vi "Demo v4_QL.vi"() -> ()   [LabVIEW 2013]
panel:
  out "0, 1":i16[](graph)
  out "Out of bound":bool
  out "Hit tube":bool
  out "Unrolled state":i32
  out "Numeric":i32
  out "Iteration":i32
  out "Q":dbl[][](array[numeric])
  in  "Slow":bool=TRUE
  out "sum":dbl
  in  "Reset Q":bool
  in  "stop":bool
  out "JUMP?":bool
  out "SCORE":i32
  out "FAIL!":bool
  in  "a":dbl=-0.3
  in  "Jump speed":dbl=3.0
  out "Picture":i32[][](graph)
  # "JUMP"
  # "FALL"
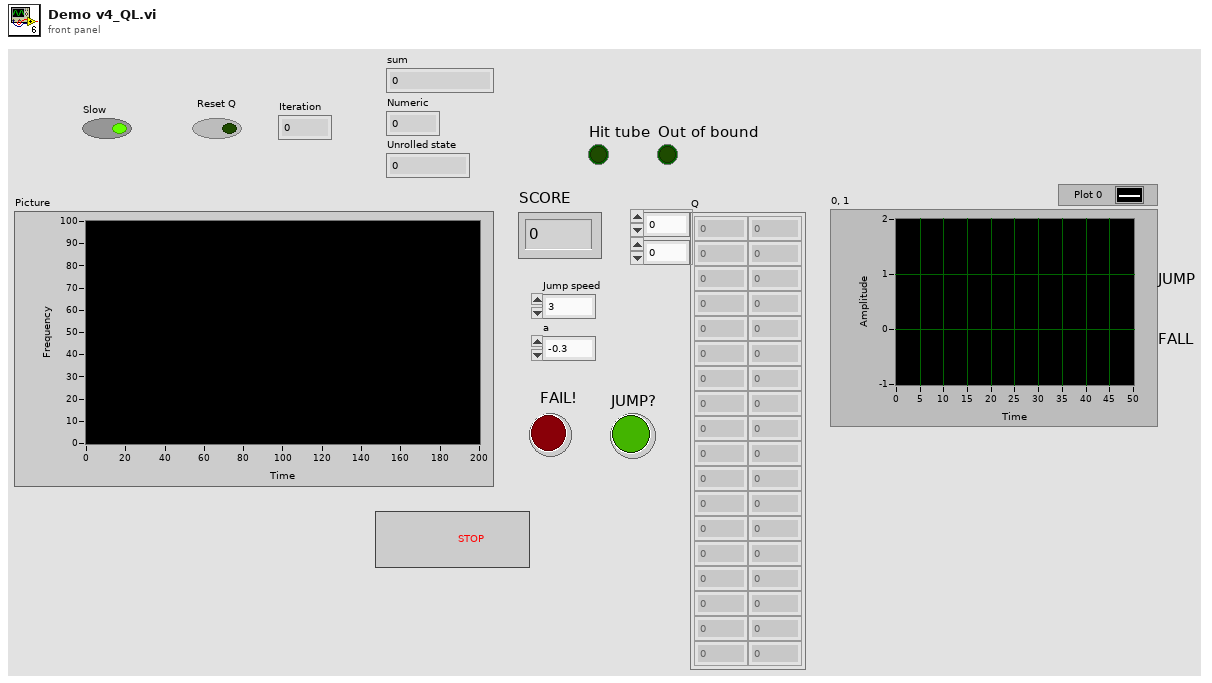
[diagram p1: front panel]
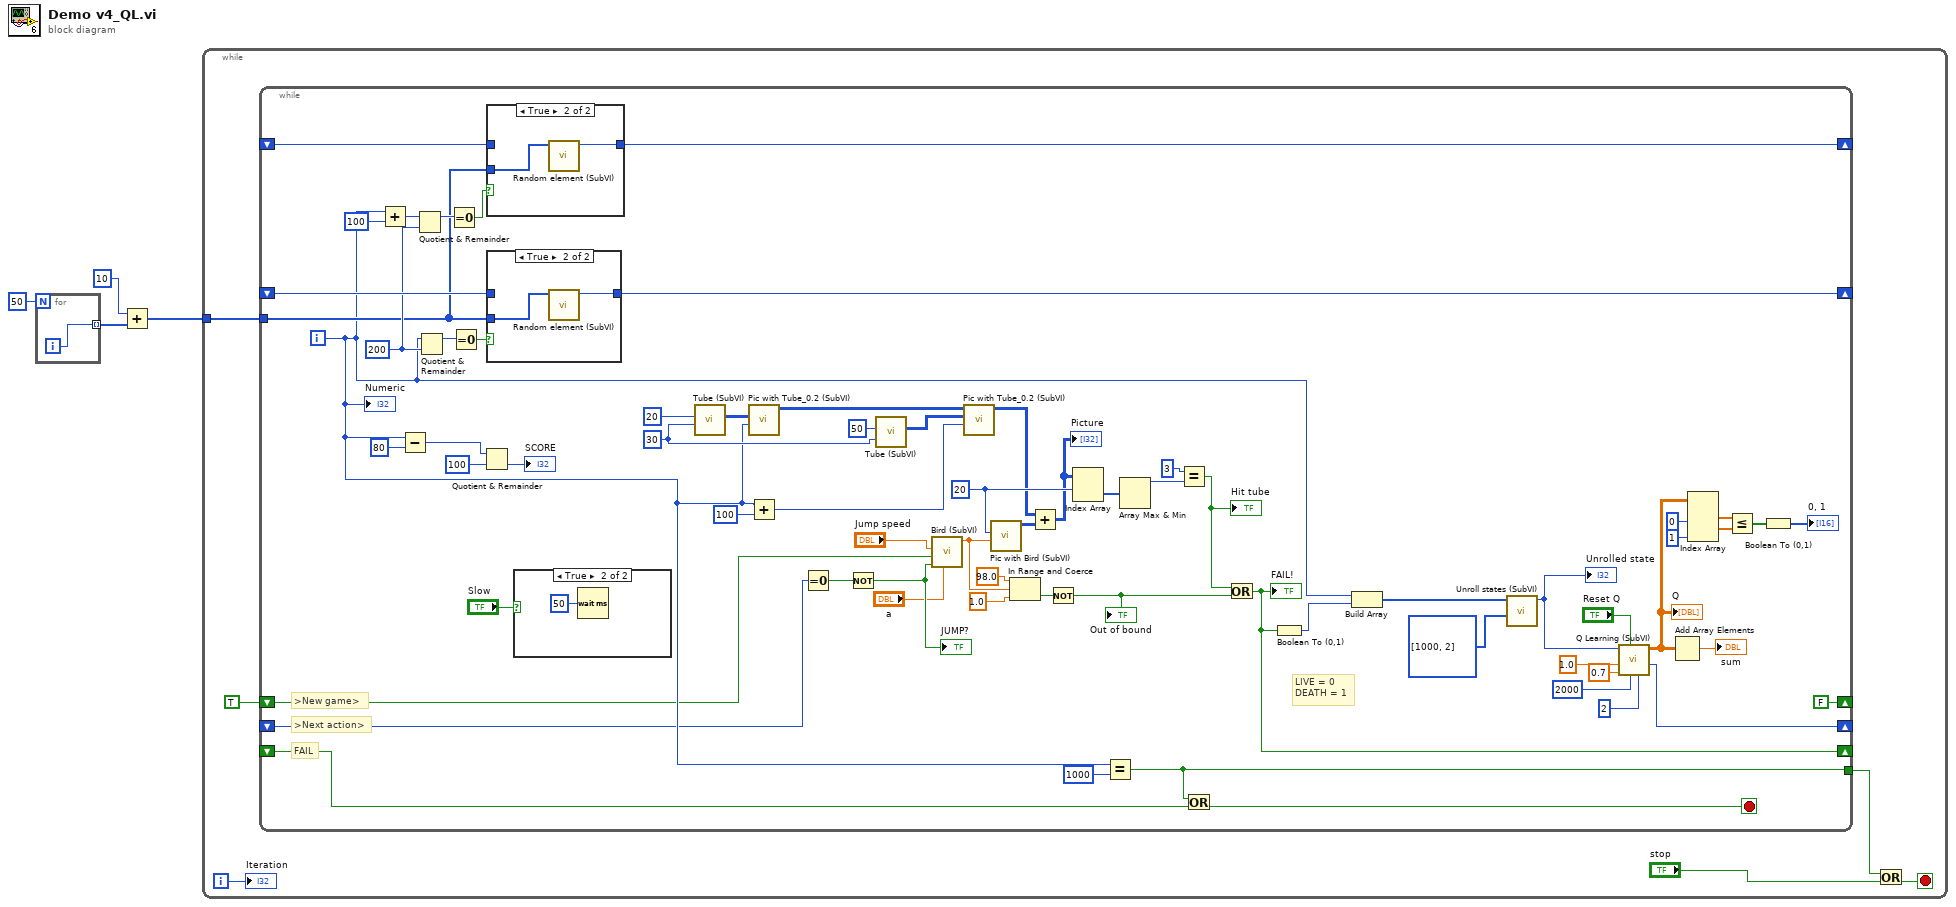
[diagram p0: block diagram]
diagram:
  n1 = for {
    N: 50 -> [_]
    tunnel: [w5] -> w3 mode=indexing
    i -> [w5]
  }
  n2 = Add(x=10, y=w3) -> (x+y=w1:i32[])
  n3 = while {
    tunnel: w1 -> [w11]
    i -> [w9]
    stop <- w8 stop-if-true
    n4 = while {
      tunnel: w11 -> [w56]
      shift-right: [w47] -> _
      shift-left: _ -> [w63]
      shift-right: [w46] -> _
      shift-left: _ -> [w57]
      shift-right: [w32] -> _
      shift-left: _ -> [w15]
      tunnel: [w27] -> w7
      shift-right: [FALSE] -> _
      shift-left: TRUE -> [w16]
      shift-right: [w13] -> _
      shift-left: _ -> [w12]
      i -> [w17]
      stop <- w28 stop-if-true
      w59 = 200 ("y")
      w68 = 20 ("X position")
      w76 = 30 ("Gap height (30)")
      # ">New game>"
      # ">Next action>"
      # "FAIL"
      # "LIVE = 0\nDEATH = 1"
      n5 = Add(x=w17, y=100) -> (x+y=w60:i32)
      n6 = Subtract(x=w17, y=80) -> (x-y=w53:i32)
      n7 = Quotient & Remainder(x=w60, y=w59) -> (x-y*floor(x/y)=w61:i32)  [unwired: 1 out]
      n8 = Quotient & Remainder(x=w17, y=w59) -> (x-y*floor(x/y)=w65:i32)  [unwired: 1 out]
      n9 = Equal To 0?(x=w61) -> (x = 0?=w58:bool)
      n10 = Equal To 0?(x=w65) -> (x = 0?=w64:bool)
      n11 = Quotient & Remainder(x=w53, y=100) -> (floor(x/y)=→"SCORE":i32)  [unwired: 1 out]
      n12 = case shown="True" w58 {
        tunnel: [w82 w84] -> w46
        tunnel: w57 -> [w82 _]
        tunnel: w56 -> [_ w83]
        frame False {
        }
        frame True {
          n13 = call "Random element (SubVI).vi"("Array"=w83) -> ("random element"=w84:i32)  [unwired: 10 in]
        }
      }
      n14 = case shown="True" w64 {
        tunnel: [w85 w87] -> w47
        tunnel: w63 -> [w85 _]
        tunnel: w56 -> [_ w86]
        frame False {
        }
        frame True {
          n15 = call "Random element (SubVI).vi"("Array"=w86) -> ("random element"=w87:i32)  [unwired: 10 in]
        }
      }
      n16 = case shown="True" "Slow" {
        frame False {
        }
        frame True {
          n17 = Wait (ms)(milliseconds to wait=u32 50) -> ()  [unwired: 1 out]
        }
      }
      n18 = call "Tube (SubVI).vi"("Gap height (30)"=w76, "Gap low y"=20) -> ("Tube"=w78:i32[][])  [unwired: 9 in]
      n19 = call "Pic with Tube_0.2 (SubVI).vi"("Tube x"=w17, "Tube"=w78) -> ("Picture"=w77:i32[][])  [unwired: 9 in]
      n20 = Add(x=w17, y=100) -> (x+y=w33:i32)
      n21 = Equal To 0?(x=w12) -> (x = 0?=w45:bool)
      n22 = Not(x=w45) -> (.not. x?=w44:bool)
      "JUMP?" <- w44
      n23 = call "Tube (SubVI).vi"("Gap height (30)"=w76, "Gap low y"=50) -> ("Tube"=w19:i32[][])  [unwired: 9 in]
      n24 = call "Bird (SubVI).vi"("a"="a", "Jump"=w44, "Reset"=w16, "Jump speed"="Jump speed") -> ("Position"=w75:dbl)  [unwired: 7 in]
      n25 = call "Pic with Tube_0.2 (SubVI).vi"("Tube x"=w33, "Tube"=w19, "Picture in"=w77) -> ("Picture"=w36:i32[][])  [unwired: 8 in]
      n26 = call "Pic with Bird (SubVI).vi"("Bird Position"=w75, "X position"=w68) -> ("Picture"=w80:i32[][])  [unwired: 9 in]
      n27 = In Range and Coerce(upper limit=98.0, x=w75, lower limit=1.0) -> (In Range?=w72:bool)  [unwired: 1 out]
      n28 = Add(x=w36, y=w80) -> (x+y=w67:i32[][])
      "Picture" <- w67
      n29 = Not(x=w72) -> (.not. x?=w66:bool)
      "Out of bound" <- w66
      n30 = Index Array(array=w67, index (row)=w68) -> (element=w71:i32[])  [unwired: 1 in]
      n31 = Equal?(x=w17, y=1000) -> (x = y?=w27:bool)
      n32 = Array Max & Min(array=w71) -> (max value=w70:i32)  [unwired: 3 out]
      n33 = Equal?(x=3 ("y"), y=w70) -> (x = y?=w37:bool)
      "Hit tube" <- w37
      n34 = Or(x=w27, y=w15) -> (x .or. y?=w28:bool)
      n35 = Or(x=w37, y=w66) -> (x .or. y?=w32:bool)
      "FAIL!" <- w32
      n36 = Boolean To (0,1)(Boolean=w32) -> (0, 1=w41:i16)
      n37 = Build Array(w17, w41) -> (w48:i32[])
      n38 = call "Unroll states (SubVI).vi"("# each state"=i32[] [1000, 2], "State array"=w48) -> ("Unrolled state"=w42:i32)  [unwired: 9 in]
      "Unrolled state" <- w42
      n39 = call "Q Learning (SubVI).vi"("# action"=2, "# state"=2000, "Reset"="Reset Q", "alpha"=0.7, "Gamma"=1.0, "State"=w42) -> ("Next Action"=w13:i32, "Q"=w26:dbl[][])  [unwired: 4 in]
      "Q" <- w26
      n40 = Add Array Elements(numeric array=w26) -> (sum=→"sum":dbl)
      n41 = Index Array(array=w26, index (col) #1=0 ("disabled index (col)"), index (col) #2=1 ("index (col)")) -> (element #1=w23:dbl[], element #2=w22:dbl[])  [unwired: 2 in]
      n42 = Less Or Equal?(x=w23, y=w22) -> (x <= y?=w21:bool[])
      n43 = Boolean To (0,1)(Boolean=w21) -> (0, 1=→"0, 1":i16[])
      "Numeric" <- w17
    }
    n44 = Or(x=w7, y="stop") -> (x .or. y?=w8:bool)
    "Iteration" <- w9
  }
